vi "SmartSEM Remote API set float.vi"(5 "wait (ms)":u32, 7 "Iterations":u32=3, 8 "error in":errorcluster, 9 "vValue":sgl, 10 "lpszParam":string, 11 "ActiveX Container":refnum<k7>(container)) -> (0 "error out":errorcluster, 3 "reference out":refnum<k7>)   [LabVIEW 2018]
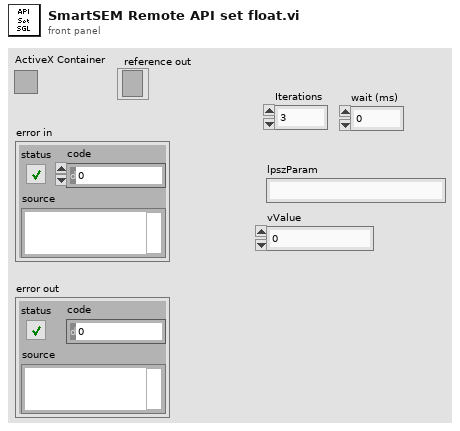
[diagram p1: front panel]
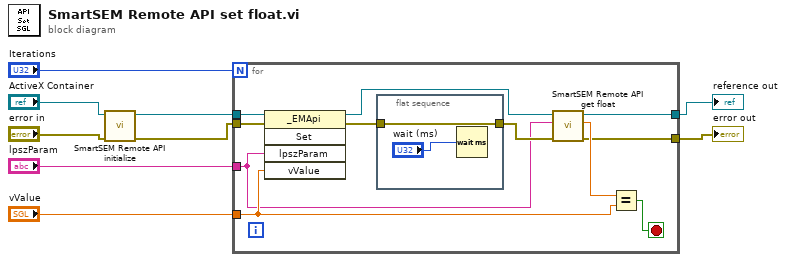
[diagram p0: block diagram]
diagram:
  n1 = call "SmartSEM Remote API initialize.vi"("error in"="error in", "ActiveX Container"="ActiveX Container") -> ("error out"=w2:errorcluster, "reference out"=w3:refnum<k7>)  [unwired: 8 in]
  n2 = for {
    N: "Iterations" -> [_]
    tunnel: w3 -> [w20]
    tunnel: w2 -> [w19]
    tunnel: [w11] -> w7
    tunnel: [w10] -> w6
    tunnel: "vValue" -> [w17]
    tunnel: "lpszParam" -> [w13]
    stop <- w18 stop-if-true
    n3 = invoke class="_EMApi" method="Set"(reference=w20, error in=w19, "lpszParam"=w13, "vValue"=w17) -> (reference out=w14:refnum<k7>, error out=w16:errorcluster)  [unwired: 1 in, 3 out]
    n4 = flat-sequence {
      tunnel: [w22] -> w15
      tunnel: w16 -> [w22]
      frame #0 {
        n5 = Wait (ms)(milliseconds to wait="wait (ms)") -> ()  [unwired: 1 out]
      }
    }
    n6 = call "SmartSEM Remote API get float.vi"("error in"=w15, "lpszParam"=w13, "ActiveX Container"=w14) -> ("error out"=w10:errorcluster, "vValue"=w12:sgl, "reference out"=w11:refnum<k7>)  [unwired: 6 in]
    n7 = Equal?(x=w12, y=w17) -> (x = y?=w18:bool)
  }
  "error out" <- w6
  "reference out" <- w7
